vi "StoreInFileNumber.vi"(0 "show path":bool, 2 "delimiter":string="\t", 3 "Enable":bool, 4 "Data":dbl[](array[numeric]), 5 "FileName":string="data", 6 "format":string="%.3f") -> (1 "Comp":bool)   [LabVIEW 2018]
uses:
  <vilib>/Utility/file.llb/Write Delimited Spreadsheet (DBL).vi
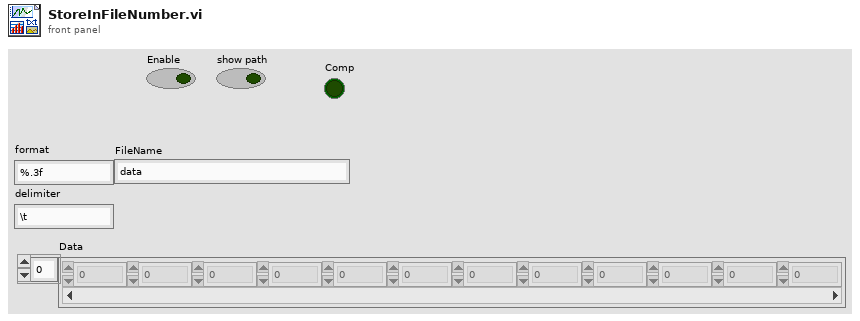
[diagram p1: front panel]
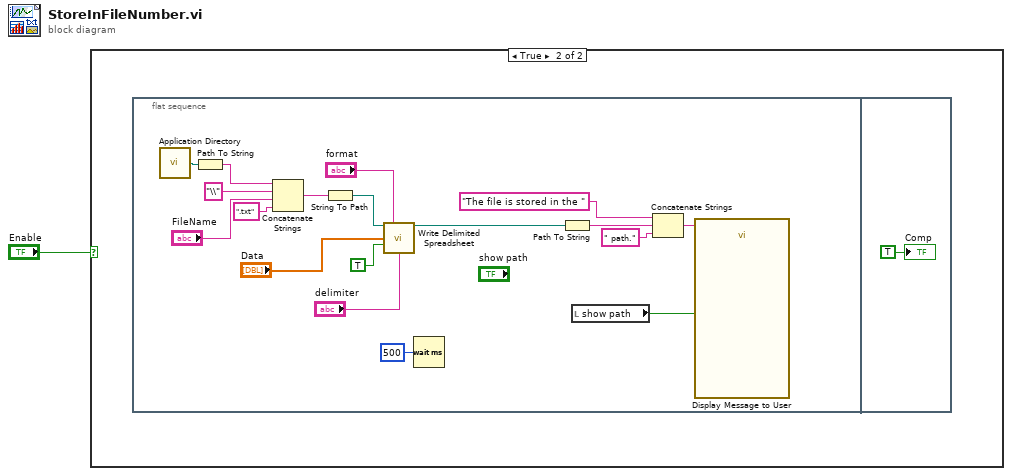
[diagram p0: block diagram]
diagram:
  n1 = case shown="True" "Enable" {
    frame False {
    }
    frame True {
      n2 = flat-sequence {
        frame #0 {
          n3 = call <vilib>:"Application Directory.vi"() -> ("Application Directory"=w11:path)
          n4 = Path To String(path=w11) -> (string=w15:string)
          n5 = Concatenate Strings(w15, "\\" ("string"), "FileName", ".txt" ("string")) -> (w18:string)
          n6 = String To Path(string=w18) -> (path=w16:path)
          n7 = call-poly <vilib>:"Write Delimited Spreadsheet.vi"("file path (dialog if empty)"=w16, "format (%.3f)"="format", "1D data"="Data", "append to file? (new file:F)"=TRUE, "delimiter (\\t)"="delimiter") -> ("new file path (Not A Path if cancelled)"=w14:path)  [unwired: 9 in, 1 out]
          n8 = Wait (ms)(milliseconds to wait=u32 500) -> ()  [unwired: 1 out]
          n9 = Path To String(path=w14) -> (string=w7:string)
          n10 = local read "show path"() -> (w4:bool)
          n11 = Concatenate Strings("The file is stored in the " ("string"), w7, " path." ("string")) -> (w6:string)
          n12 = call "Display Message to User"("Enable"=w4, "Message"=w6) -> ()  [unwired: 8 in, 2 out]
        }
        frame #1 {
          "Comp" <- TRUE ("comp")
        }
      }
    }
  }
